vi "FMDLKeithley6514InitiateImmediateReadDataClearBufferRearmTrigger.vi"(0 "VISA resource name":refnum<visa-resource-name>, 1 "Arm Source (1: Immediate)":i32(ring)=1 items=["Hold", "Immediate", "Real-time Clock", "Manual", "Bus", "Trigger Link", "External Triggering", "Timer", "STest", "PSTest", "NSTest", "BSTest"], 2 "OD3 engaged on 918D?":bool, 3 "Arm Count (1)":i32=1, 4 "Arm Timer Interval (0.1 s)":dbl=0.1, 5 "error in (no error)":errorcluster, 6 "Timeout (10000 ms)":u32=10000, 7 "Buffer size previously set":i32) -> (10 "Number of times the loop ran":i32, 11 "Number of Readings in K6514 Buffer":i32, 12 "Maximum":dbl, 13 "Minimum":dbl, 14 "VISA resource name out":refnum<visa-resource-name>, 15 "Mean":dbl, 17 "Standard Deviation":dbl, 18 "Peak-to-Peak":dbl, 19 "error out":errorcluster)   [LabVIEW 2018]
uses:
  <instrlib>/Keithley 6517/Keithley 6517.lvlib
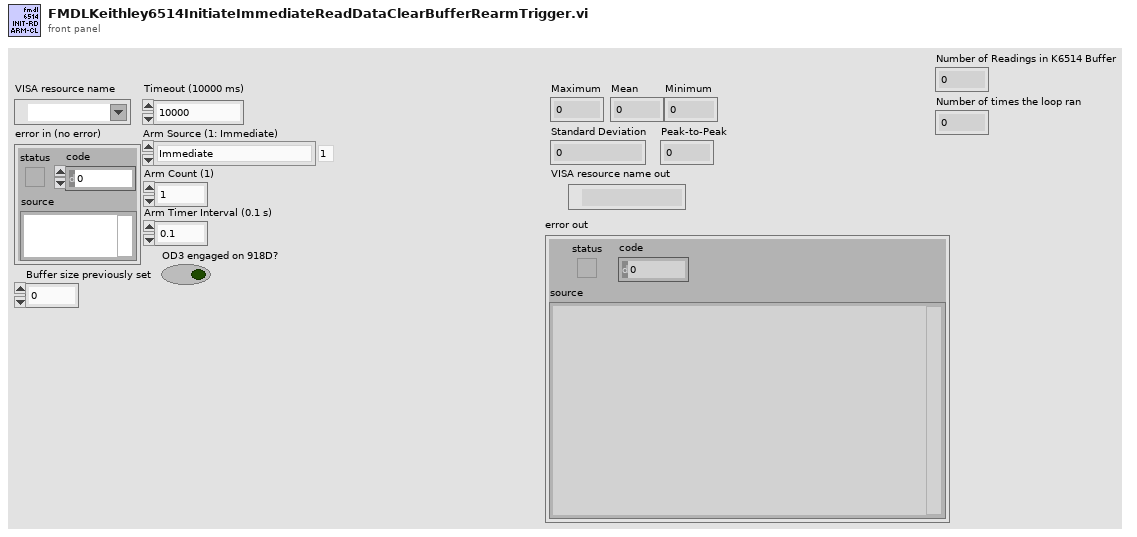
[diagram p1: front panel]
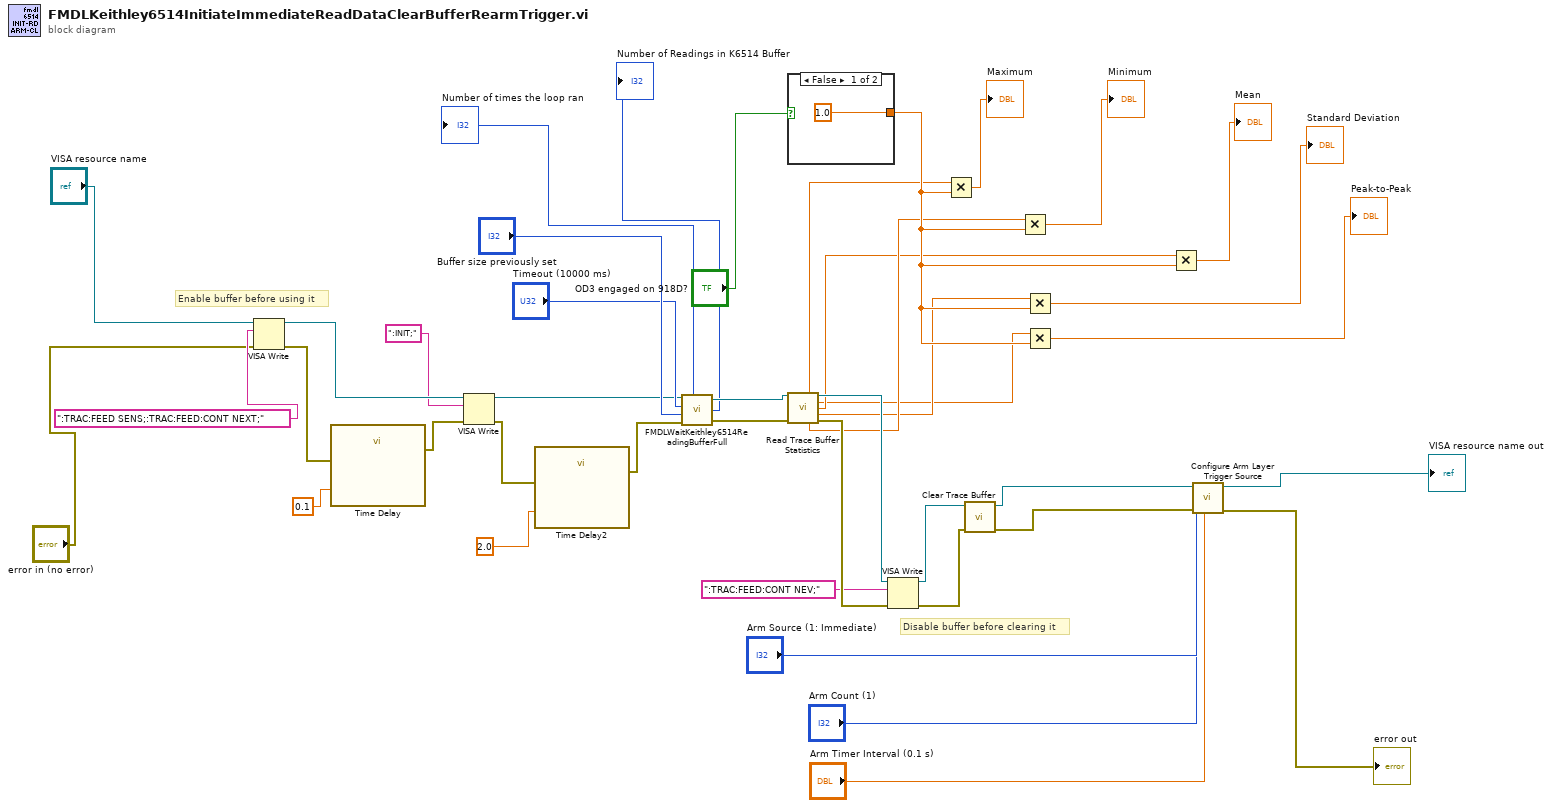
[diagram p0: block diagram]
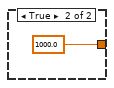
[diagram p2: hidden frame]
diagram:
  # "Enable buffer before using it"
  # "Disable buffer before clearing it"
  n1 = VISA Write(VISA resource name="VISA resource name", write buffer=":TRAC:FEED SENS;:TRAC:FEED:CONT NEXT;" ("true string"), error in (no error)="error in (no error)") -> (VISA resource name out=w17:refnum<visa-resource-name>, error out=w28:errorcluster)  [unwired: 1 out]
  n2 = call "Time Delay"("error in (no error)"=w28, "Delay Time (s)"=0.1) -> ("error out"=w16:errorcluster)  [unwired: 9 in]
  n3 = VISA Write(VISA resource name=w17, write buffer=":INIT;", error in (no error)=w16) -> (VISA resource name out=w15:refnum<visa-resource-name>, error out=w14:errorcluster)  [unwired: 1 out]
  n4 = call "Time Delay2"("error in (no error)"=w14, "Delay Time (s)"=2.0) -> ("error out"=w21:errorcluster)  [unwired: 9 in]
  n5 = call "FMDLWaitKeithley6514ReadingBufferFull.vi"("VISA resource name"=w15, "Timeout (10000 ms)"="Timeout (10000 ms)", "Buffer size previously set"="Buffer size previously set", "error in (no error)"=w21) -> ("Number of times the loop ran"=→"Number of times the loop ran":i32, "VISA resource name out"=w36:refnum<visa-resource-name>, "Number of Readings in Buffer"=→"Number of Readings in K6514 Buffer":i32, "error out"=w26:errorcluster)
  n6 = case shown="False" "OD3 engaged on 918D?" {
    tunnel: [1.0 1000.0] -> w11
    frame False {
    }
    frame True {
    }
  }
  n7 = call <instrlib>:"Read Trace Buffer Statistics.vi"("VISA resource name"=w36, "error in (no error)"=w26) -> ("Maximum"=w10:dbl, "VISA resource name out"=w35:refnum<visa-resource-name>, "Peak-to-Peak"=w2:dbl, "Mean"=w6:dbl, "Standard Deviation"=w4:dbl, "Minimum"=w8:dbl, "error out"=w33:errorcluster)  [unwired: 7 in]
  n8 = VISA Write(VISA resource name=w35, write buffer=":TRAC:FEED:CONT NEV;" ("true string"), error in (no error)=w33) -> (VISA resource name out=w34:refnum<visa-resource-name>, error out=w29:errorcluster)  [unwired: 1 out]
  n9 = Multiply(x=w10, y=w11) -> (x*y=→"Maximum":dbl)
  n10 = call <instrlib>:"Clear Trace Buffer.vi"("error in (no error)"=w29, "VISA resource name"=w34) -> ("error out"=w30:errorcluster, "VISA resource name out"=w42:refnum<visa-resource-name>)  [unwired: 8 in]
  n11 = Multiply(x=w8, y=w11) -> (x*y=→"Minimum":dbl)
  n12 = Multiply(x=w4, y=w11) -> (x*y=→"Standard Deviation":dbl)
  n13 = Multiply(x=w2, y=w11) -> (x*y=→"Peak-to-Peak":dbl)
  n14 = Multiply(x=w6, y=w11) -> (x*y=→"Mean":dbl)
  n15 = call <instrlib>:"Configure Arm Layer Trigger Source.vi"("Arm Timer Interval (0.1 s)"="Arm Timer Interval (0.1 s)", "error in (no error)"=w30, "Arm Count (1)"="Arm Count (1)", "Arm Source (1: Immediate)"="Arm Source (1: Immediate)", "VISA resource name"=w42) -> ("error out"=→"error out":errorcluster, "VISA resource name out"=→"VISA resource name out":refnum<visa-resource-name>)  [unwired: 5 in]
